vi "Language to Abbreviation.vi"(8 "error in (no error)":errorcluster, 11 "Language":T1) -> (0 "error out":errorcluster, 3 "Language Abbreviation":string)   [LabVIEW 2017, in "Dark Sky Weather Data for LabVIEW.lvlib"]
doc: "Accepts the language enum, which lists languages in plain text, and converts to the language value needed by the Dark Sky API."
uses:
  Dark Sky Weather Data for LabVIEW.lvlib
  Controls/Language Enum.ctl
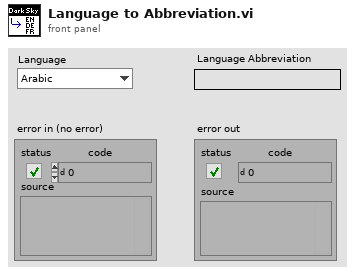
[diagram p1: front panel]
types:
  T1 = typedef "Dark Sky Weather Data for LabVIEW.lvlib/Language Enum.ctl" = enum16{"Arabic", "Azerbaijani", "Belaursian", "Bulgarian", "Bosnian", "Catalan", "Czech", "German", "Greek", "English", "Spanish", "Estonian", "French", "Croatian", "Hungarian", "Indonesian", "Italian", "Icelandic", "Georgian", "Cornish", "Norwegian Bokmal", "Dutch", "Polish", "Portuguese", "Russian", "Slovak", "Slovenian", "Serbian", "Swedish", "Tetum", "Turkish", "Ukrainian", "simplified Chinese", "traditional Chinese"}
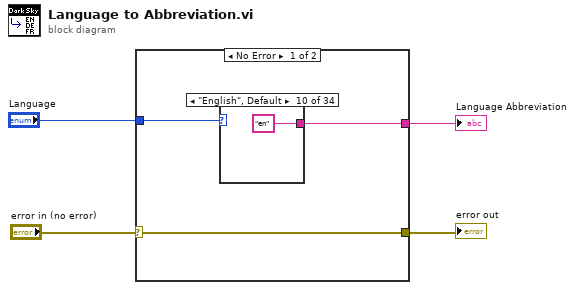
[diagram p0: block diagram]
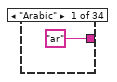
[diagram p2: hidden frame]
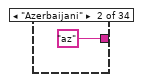
[diagram p3: hidden frame]
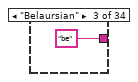
[diagram p4: hidden frame]
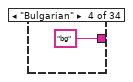
[diagram p5: hidden frame]
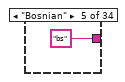
[diagram p6: hidden frame]
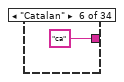
[diagram p7: hidden frame]
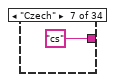
[diagram p8: hidden frame]
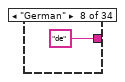
[diagram p9: hidden frame]
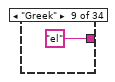
[diagram p10: hidden frame]
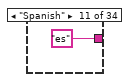
[diagram p11: hidden frame]
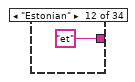
[diagram p12: hidden frame]
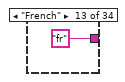
[diagram p13: hidden frame]
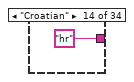
[diagram p14: hidden frame]
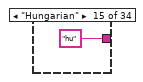
[diagram p15: hidden frame]
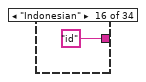
[diagram p16: hidden frame]
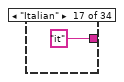
[diagram p17: hidden frame]
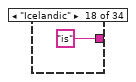
[diagram p18: hidden frame]
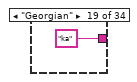
[diagram p19: hidden frame]
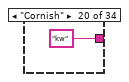
[diagram p20: hidden frame]
diagram:
  n1 = case shown="No Error" "error in (no error)" {
    selector: "error in (no error)" -> [w5 w43]
    tunnel: "Language" -> [w7 _]
    tunnel: [w6 "en"] -> w2
    tunnel: [w5 w43] -> w1
    frame No Error {
      n2 = case shown="\"English\", Default" w7 {
        tunnel: ["ar" "az" "be" "bg" "bs" "ca" "cs" "de" "el" "en" "es" "et" "fr" "hr" "hu" "id" "it" "is" "ka" "kw" "nb" "nl" "pl" "pt" "ru" "sk" "sl" "sr" "sv" "tet" "tr" "uk" "zh" "zh-tw"] -> w6
        frame "Arabic" {
        }
        frame "Azerbaijani" {
        }
        frame "Belaursian" {
        }
        frame "Bulgarian" {
        }
        frame "Bosnian" {
        }
        frame "Catalan" {
        }
        frame "Czech" {
        }
        frame "German" {
        }
        frame "Greek" {
        }
        frame "English", Default {
        }
        frame "Spanish" {
        }
        frame "Estonian" {
        }
        frame "French" {
        }
        frame "Croatian" {
        }
        frame "Hungarian" {
        }
        frame "Indonesian" {
        }
        frame "Italian" {
        }
        frame "Icelandic" {
        }
        frame "Georgian" {
        }
        frame "Cornish" {
        }
        frame "Norwegian Bokmal" {
        }
        frame "Dutch" {
        }
        frame "Polish" {
        }
        frame "Portuguese" {
        }
        frame "Russian" {
        }
        frame "Slovak" {
        }
        frame "Slovenian" {
        }
        frame "Serbian" {
        }
        frame "Swedish" {
        }
        frame "Tetum" {
        }
        frame "Turkish" {
        }
        frame "Ukrainian" {
        }
        frame "simplified Chinese" {
        }
        frame "traditional Chinese" {
        }
      }
    }
    frame Error {
    }
  }
  "Language Abbreviation" <- w2
  "error out" <- w1
